vi "8CHDAQ - Save Data File.vi"(9 "Array":dbl[][](array[numeric]), 10 "Sampling Rate":dbl, 11 "Channel Data":T1) -> ()   [LabVIEW 2015]
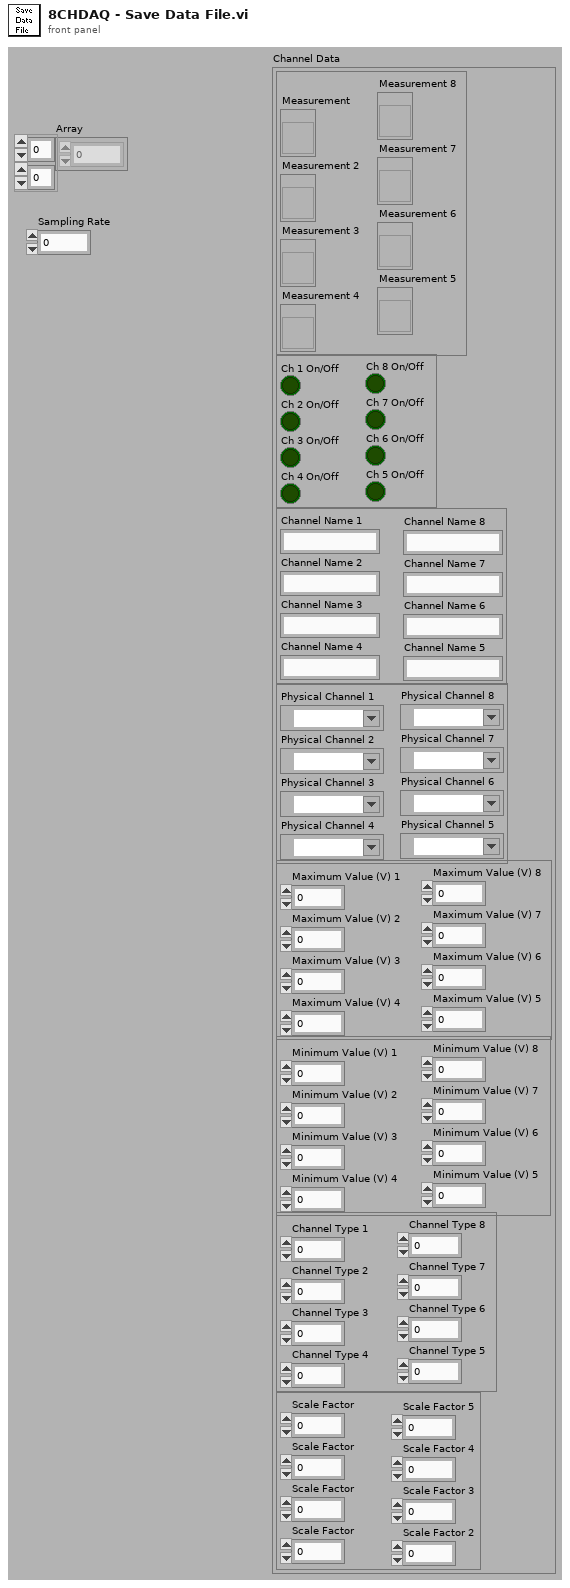
[diagram p1: front panel]
types:
  T1 = cluster{cluster{"Measurement":refnum<vi>, "Measurement 2":refnum<vi>, "Measurement 3":refnum<vi>, "Measurement 4":refnum<vi>, "Measurement 5":refnum<vi>, "Measurement 6":refnum<vi>, "Measurement 7":refnum<vi>, "Measurement 8":refnum<vi>}, cluster{"Ch 1 On/Off":bool, "Ch 2 On/Off":bool, "Ch 3 On/Off":bool, "Ch 4 On/Off":bool, "Ch 5 On/Off":bool, "Ch 6 On/Off":bool, "Ch 7 On/Off":bool, "Ch 8 On/Off":bool}, cluster{"Channel Name 1":string, "Channel Name 2":string, "Channel Name 3":string, "Channel Name 4":string, "Channel Name 5":string, "Channel Name 6":string, "Channel Name 7":string, "Channel Name 8":string}, cluster{"Physical Channel 1":tag, "Physical Channel 2":tag, "Physical Channel 3":tag, "Physical Channel 4":tag, "Physical Channel 5":tag, "Physical Channel 6":tag, "Physical Channel 7":tag, "Physical Channel 8":tag}, cluster{"Maximum Value (V) 1":dbl, "Maximum Value (V) 2":dbl, "Maximum Value (V) 3":dbl, "Maximum Value (V) 4":dbl, "Maximum Value (V) 5":dbl, "Maximum Value (V) 6":dbl, "Maximum Value (V) 7":dbl, "Maximum Value (V) 8":dbl}, cluster{"Minimum Value (V) 1":dbl, "Minimum Value (V) 2":dbl, "Minimum Value (V) 3":dbl, "Minimum Value (V) 4":dbl, "Minimum Value (V) 5":dbl, "Minimum Value (V) 6":dbl, "Minimum Value (V) 7":dbl, "Minimum Value (V) 8":dbl}, cluster{"Channel Type 1":u16, "Channel Type 2":u16, "Channel Type 3":u16, "Channel Type 4":u16, "Channel Type 5":u16, "Channel Type 6":u16, "Channel Type 7":u16, "Channel Type 8":u16}, cluster{"Scale Factor":dbl[unit], "Scale Factor":dbl[unit], "Scale Factor":dbl[unit], "Scale Factor":dbl[unit], "Scale Factor 2":dbl[unit], "Scale Factor 3":dbl[unit], "Scale Factor 4":dbl[unit], "Scale Factor 5":dbl[unit]}}
  T2 = enum16{"open", "replace", "create", "open or create", "replace or create", "replace or create with confirmation"}
  T3 = cluster{"Ch 1 On/Off":bool, "Ch 2 On/Off":bool, "Ch 3 On/Off":bool, "Ch 4 On/Off":bool, "Ch 5 On/Off":bool, "Ch 6 On/Off":bool, "Ch 7 On/Off":bool, "Ch 8 On/Off":bool}
  T4 = cluster{"Channel Name 1":string, "Channel Name 2":string, "Channel Name 3":string, "Channel Name 4":string, "Channel Name 5":string, "Channel Name 6":string, "Channel Name 7":string, "Channel Name 8":string}
  T5 = cluster{"Channel Type 1":u16, "Channel Type 2":u16, "Channel Type 3":u16, "Channel Type 4":u16, "Channel Type 5":u16, "Channel Type 6":u16, "Channel Type 7":u16, "Channel Type 8":u16}
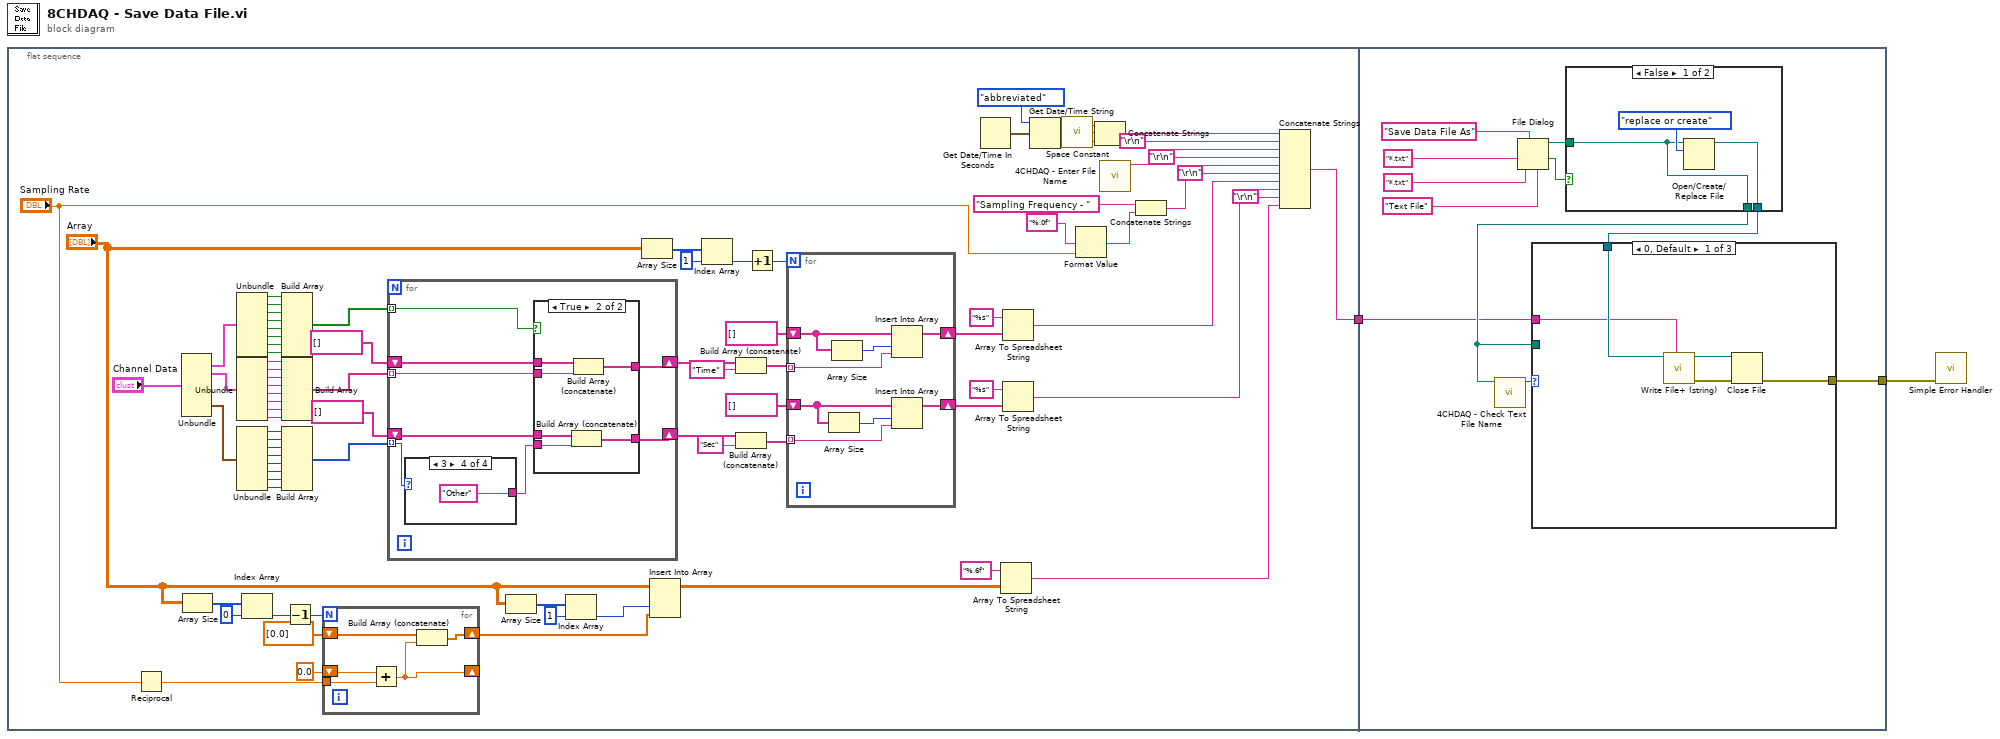
[diagram p0: block diagram]
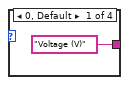
[diagram p2: hidden frame]
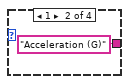
[diagram p3: hidden frame]
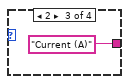
[diagram p4: hidden frame]
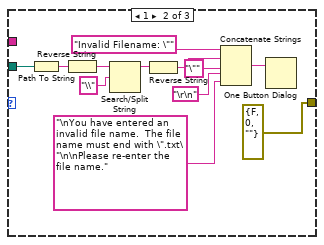
[diagram p6: hidden frame]
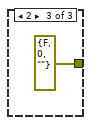
[diagram p7: hidden frame]
diagram:
  n1 = flat-sequence {
    tunnel: [w46] -> w2
    tunnel: w2 -> [w121]
    tunnel: [w119] -> w1
    frame #0 {
      n2 = Reciprocal(x="Sampling Rate") -> (1/x=w34:dbl)
      n3 = Unbundle("Channel Data") -> (w83:T3, w68:T4, w69:T5)  [unwired: 5 out]
      n4 = Array Size(array="Array") -> (size(s)=w36:i32[])
      n5 = Unbundle(w83) -> ("Ch 1 On/Off"=w82:bool, "Ch 2 On/Off"=w81:bool, "Ch 3 On/Off"=w80:bool, "Ch 4 On/Off"=w79:bool, "Ch 5 On/Off"=w14:bool, "Ch 6 On/Off"=w13:bool, "Ch 7 On/Off"=w12:bool, "Ch 8 On/Off"=w11:bool)
      n6 = Unbundle(w68) -> ("Channel Name 1"=w74:string, "Channel Name 2"=w75:string, "Channel Name 3"=w76:string, "Channel Name 4"=w77:string, "Channel Name 5"=w9:string, "Channel Name 6"=w10:string, "Channel Name 7"=w7:string, "Channel Name 8"=w8:string)
      n7 = Unbundle(w69) -> ("Channel Type 1"=w73:u16, "Channel Type 2"=w72:u16, "Channel Type 3"=w71:u16, "Channel Type 4"=w70:u16, "Channel Type 5"=w3:u16, "Channel Type 6"=w4:u16, "Channel Type 7"=w5:u16, "Channel Type 8"=w6:u16)
      n8 = Index Array(array=w36, index=0) -> (element=w32:i32)
      n9 = Build Array(w82, w81, w80, w79, w14, w13, w12, w11) -> (w78:bool[])
      n10 = Build Array(w74, w75, w76, w77, w9, w10, w7, w8) -> (w67:string[])
      n11 = Build Array(w73, w72, w71, w70, w3, w4, w5, w6) -> (w66:u16[])
      n12 = Decrement(x=w32) -> (x-1=w31:i32)
      n13 = for {
        N: w31 -> [_]
        tunnel: w34 -> [w90]
        shift-right: [w88] -> _
        shift-left: 0.0 -> [w89]
        shift-right: [w87] -> w16
        shift-left: dbl[] [0.0] -> [w86]
        n14 = Add(x=w89, y=w90) -> (x+y=w88:dbl)
        n15 = Build Array (concatenate)(w86, w88) -> (w87:dbl[])
      }
      n16 = for {
        tunnel: w78 -> [w98] mode=indexing
        tunnel: w67 -> [w97] mode=indexing
        tunnel: w66 -> [w94] mode=indexing
        shift-right: [w96] -> w22
        shift-left: string[] [] -> [w95]
        shift-right: [w92] -> w20
        shift-left: string[] [] -> [w91]
        n17 = case shown="3" w94 {
          tunnel: ["Voltage (V)" "Acceleration (G)" "Current (A)" "Other"] -> w93
          frame 0, Default {
          }
          frame 1 {
          }
          frame 2 {
          }
          frame 3 {
          }
        }
        n18 = case shown="True" w98 {
          tunnel: w97 -> [_ w110]
          tunnel: [w104 w109] -> w96
          tunnel: w95 -> [w104 w108]
          tunnel: w93 -> [_ w107]
          tunnel: [w103 w106] -> w92
          tunnel: w91 -> [w103 w105]
          frame False {
          }
          frame True {
            n19 = Build Array (concatenate)(w105, w107) -> (w106:string[])
            n20 = Build Array (concatenate)(w108, w110) -> (w109:string[])
          }
        }
      }
      n21 = Array Size(array="Array") -> (size(s)=w28:i32[])
      n22 = Index Array(array=w28, index=1) -> (element=w25:i32)
      n23 = Array Size(array="Array") -> (size(s)=w85:i32[])
      n24 = Insert Into Array(array="Array", index (col)=w25, new element=w16) -> (w29:dbl[][])  [unwired: 1 in]
      n25 = Index Array(array=w85, index=1) -> (element=w17:i32)
      n26 = Build Array (concatenate)(w22, "Time") -> (w21:string[])
      n27 = Build Array (concatenate)(w20, "Sec") -> (w19:string[])
      n28 = Increment(x=w17) -> (x+1=w18:i32)
      n29 = for {
        N: w18 -> [_]
        tunnel: w21 -> [w117] mode=indexing
        shift-right: [w116] -> w61
        shift-left: string[] [] -> [w115]
        tunnel: w19 -> [w114] mode=indexing
        shift-right: [w112] -> w58
        shift-left: string[] [] -> [w111]
        n30 = Array Size(array=w111) -> (size(s)=w113:i32)
        n31 = Array Size(array=w115) -> (size(s)=w118:i32)
        n32 = Insert Into Array(array=w115, index=w118, new element=w117) -> (w116:string[])
        n33 = Insert Into Array(array=w111, index=w113, new element=w114) -> (w112:string[])
      }
      n34 = Get Date/Time In Seconds() -> (seconds since 1Jan1904=w57:timestamp)
      n35 = Array To Spreadsheet String(array=w29, 3:"%.6f" ("format string")) -> (spreadsheet string=w39:string)  [unwired: 1 in]
      n36 = Array To Spreadsheet String(array=w61, 3:"%s" ("format string")) -> (spreadsheet string=w48:string)  [unwired: 1 in]
      n37 = Array To Spreadsheet String(array=w58, 3:"%s" ("format string")) -> (spreadsheet string=w40:string)  [unwired: 1 in]
      n38 = Get Date/Time String(date format (0)=enum16{"short", "long", "abbreviated"}."abbreviated", seconds (now)=w57) -> (date string=w55:string, time string=w45:string)  [unwired: 1 in]
      n39 = call <vilib>:"Space Constant.vi"() -> ("String"=w44:string)
      n40 = Format Value(format string="%.0f", value (0)="Sampling Rate") -> (output string=w51:string)  [unwired: 1 in]
      n41 = Concatenate Strings(w55, w44, w45) -> (w54:string)
      n42 = call "4CHDAQ - Enter File Name.vi"() -> ("String 2"=w53:string)  [unwired: 11 in]
      n43 = Concatenate Strings("Sampling Frequency - ", w51) -> (w49:string)
      n44 = Concatenate Strings(w54, "\r\n", w53, "\r\n", w49, "\r\n", w48, w40, "\r\n", w39) -> (w46:string)
    }
    frame #1 {
      n45 = File Dialog(4:"Text File" ("pattern label"), 6:"*.txt" ("pattern"), 7:"Save Data File As" ("prompt"), 9:"*.txt" ("default name")) -> (1:w124:bool, 3:w125:path)  [unwired: 3 in, 2 out]
      n46 = case shown="False" w124 {
        tunnel: w125 -> [w148 w151]
        tunnel: [w148 w151] -> w122
        tunnel: [w149 _] -> w120
        frame False {
          n47 = Open/Create/Replace File(file path (use dialog)=w148, operation (0:open)=T2."replace or create") -> (refnum out=w149:refnum<file>)  [unwired: 4 in, 2 out]
        }
        frame True {
        }
      }
      n48 = call "4CHDAQ - Check Text File Name.vi"("path"=w122) -> ("Error Type"=w123:i32)  [unwired: 10 in]
      n49 = case shown="0, Default" w123 {
        tunnel: w120 -> [w134 _ _]
        tunnel: w122 -> [_ w136 _]
        tunnel: w121 -> [w133 _ _]
        tunnel: [w130 errorcluster {"status"=FALSE, "code"=0, "source"=""} ("error out") errorcluster {"status"=FALSE, "code"=0, "source"=""} ("error out")] -> w119
        frame 0, Default {
          n50 = call <vilib>:"Write File+ (string).vi"("string"=w133, "refnum"=w134) -> ("error out"=w132:errorcluster, "dup refnum"=w131:refnum<file>)  [unwired: 5 in, 1 out]
          n51 = Close File(refnum=w131, error in=w132) -> (error out=w130:errorcluster)  [unwired: 1 out]
        }
        frame 1 {
          n52 = Path To String(path=w136) -> (string=w145:string)
          n53 = Reverse String(1:w145) -> (0:w144:string)
          n54 = Search/Split String(string=w144, search string/char (-)="\\") -> (substring before match=w141:string)  [unwired: 1 in, 2 out]
          n55 = Reverse String(1:w141) -> (0:w140:string)
          n56 = Concatenate Strings("Invalid Filename: \"" ("string"), w140, "\"" ("string"), "\r\n", "\nYou have entered an invalid file name.  The file name must end with \".txt\"\n\nPlease re-enter the file name." ("message")) -> (w137:string)
          n57 = One Button Dialog(message=w137) -> ()  [unwired: 1 in, 1 out]
        }
        frame 2 {
        }
      }
    }
  }
  n58 = call <vilib>:"Simple Error Handler.vi"("error in (no error)"=w1) -> ()  [unwired: 4 in, 5 out]
